vi "Get All Aliases.vi"(8 "error in (no error)":errorcluster, 11 "Aliases Ref in":T2 format="%.0x") -> (0 "error out":errorcluster, 2 "Alias Mappings":T1[](array[typedef]), 3 "Aliases Ref out":T2 format="%.0x")   [LabVIEW 2017, in "Switch Scripting.lvlib"]
uses:
  Switch Scripting.lvlib
  <vilib>/NI Veristand/Custom Device API/Custom Device Item Ref.ctl
  Shared/Alias Mapping.ctl
  <vilib>/NI VeriStand/Custom Device API/Custom Device API.lvlib
  Shared/Routing and Faulting Shared.lvlib
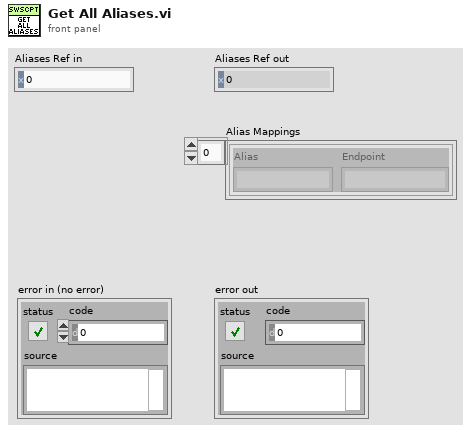
[diagram p1: front panel]
types:
  T1 = typedef "Routing and Faulting Shared.lvlib/Alias Mapping.ctl" = cluster{"Alias":string, "Endpoint":string}
  T2 = typedef "Custom Device API.lvlib/Custom Device Item Ref.ctl" = u64
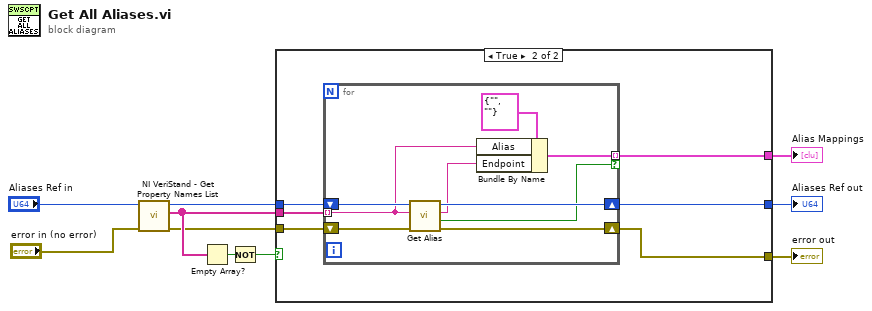
[diagram p0: block diagram]
diagram:
  n1 = call <vilib>:"NI VeriStand - Get Property Names List.vi"("error in (no error)"="error in (no error)", "Item Ref in"="Aliases Ref in") -> ("error out"=w8:errorcluster, "Property Names"=w9:string[], "Item Ref out"=w4:T2)  [unwired: 7 in]
  n2 = Empty Array?(array=w9) -> (empty?=w10:bool)
  n3 = Not(x=w10) -> (.not. x?=w2:bool)
  n4 = case shown="True" w2 {
    tunnel: w9 -> [_ w18]
    tunnel: w8 -> [w11 w17]
    tunnel: [w11 w16] -> w6
    tunnel: w4 -> [w12 w15]
    tunnel: [w12 w14] -> w3
    tunnel: [_ w13] -> w1
    frame False {
    }
    frame True {
      n5 = for {
        tunnel: w18 -> [w21] mode=indexing
        shift-right: [w24] -> w16
        shift-left: w17 -> [w25]
        tunnel: [w19] -> w13 mode=indexing if=w23
        shift-right: [w26] -> w14
        shift-left: w15 -> [w27]
        n6 = call "Get Alias.vi"("error in (no error)"=w25, "Alias"=w21, "Aliases Ref in"=w27) -> ("error out"=w24:errorcluster, "Alias found"=w23:bool, "Pin"=w20:string, "Aliases Ref out"=w26:T2)  [unwired: 5 in]
        n7 = Bundle By Name(cluster=T1 {"Alias"="", "Endpoint"=""} ("Alias Mapping"), "Alias"=w21, "Endpoint"=w20) -> (w19:T1)
      }
    }
  }
  "error out" <- w6
  "Aliases Ref out" <- w3
  "Alias Mappings" <- w1
